vi "LabVIEW MIDI Keyboard.vi"() -> ()   [LabVIEW 2016]
doc: "This example simulates a General MIDI (GM) keyboard. Use the computer keys to play the general MIDI sound you select. The example uses Event structures to get the keyboard events and a Call Library Function Node to send the MIDI messages to Windows."
panel:
  in  "?":bool
  in  "Config":bool
  in  "Help":bool
  in  "stop":bool
  in  "General MIDI instrument patch":i32(listbox)
  in  "Volume":i32(knob)=110 min=0 max=127 step=1 scale=0.0..127.0
  in  "uDeviceID":i32=1
  in  "Midi channel":i32
  # "Select Help»Show Context Help and move the cursor over the VI icon to display help for this VI."
  # "Instructions:\n1. Run the VI.\n2. Select a sound type from the General MIDI instrument patch listbox.\n3. Press a key on the computer keyboard that corresponds to a key on the image of the MIDI keyboard.\n\nNOTE: If you do not hear a sound, click the Config button to change the MIDI device number. Refer to the Windows Device Manager to determine the correct MIDI device number.\n\n4. To stop the VI, click the Stop button or press the <Esc> key."
  # "Use myRio to get the note values ?"
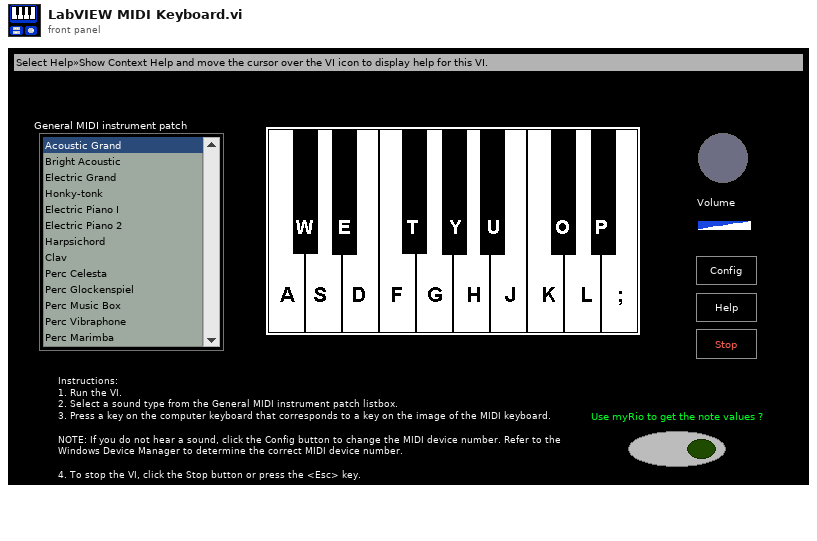
[diagram p1: front panel]
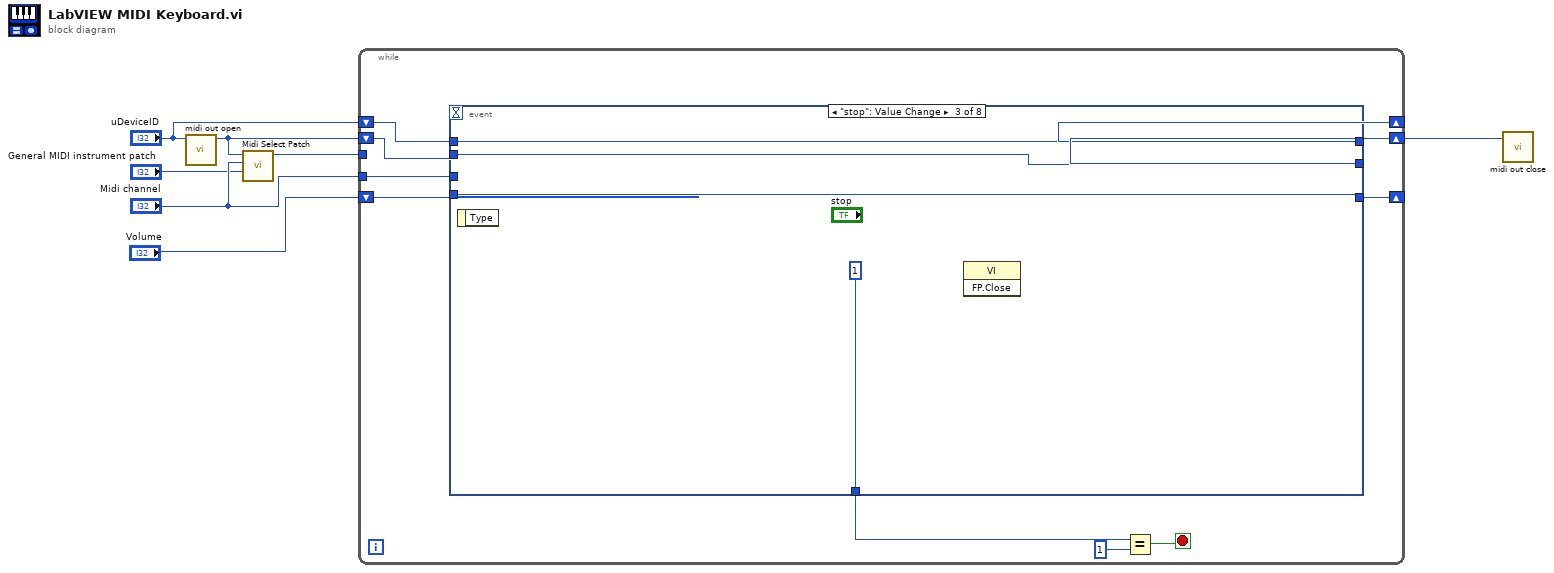
[diagram p0: block diagram]
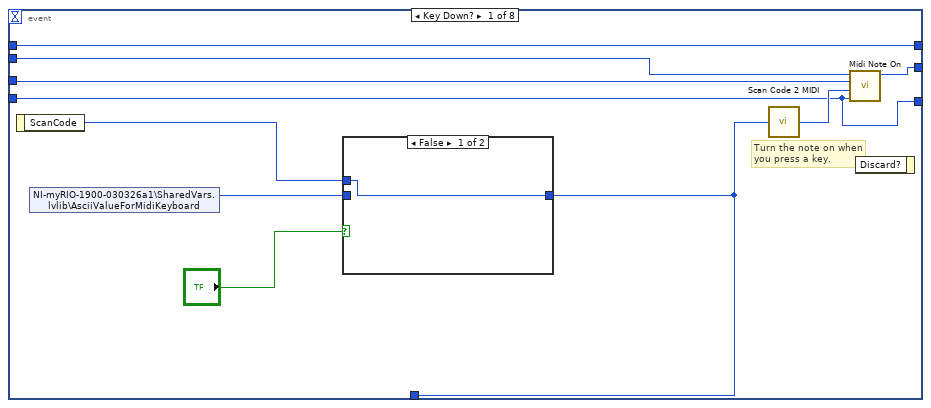
[diagram p2: hidden frame]
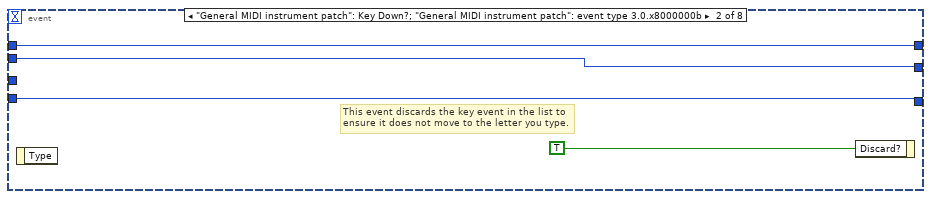
[diagram p4: hidden frame]
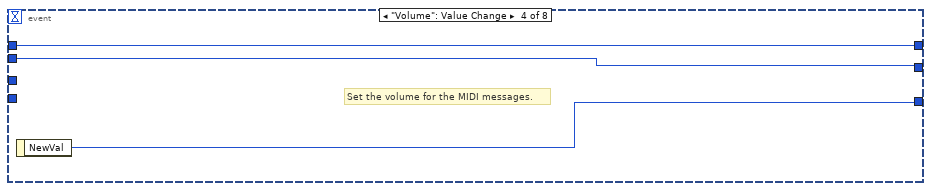
[diagram p5: hidden frame]
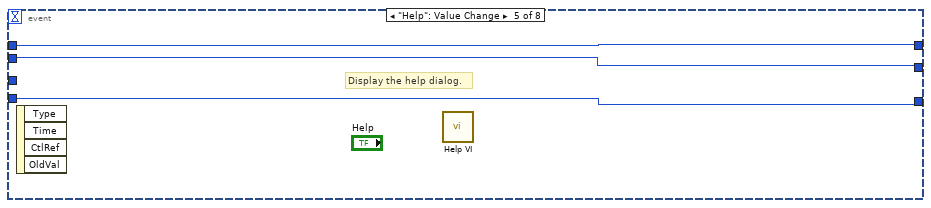
[diagram p6: hidden frame]
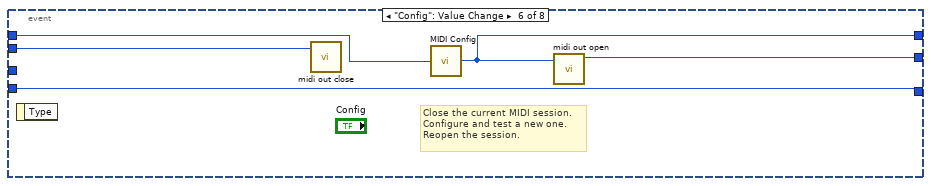
[diagram p7: hidden frame]
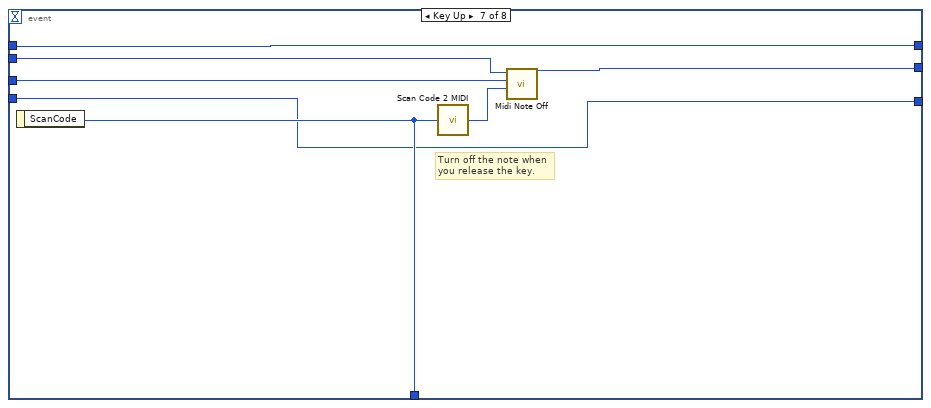
[diagram p8: hidden frame]
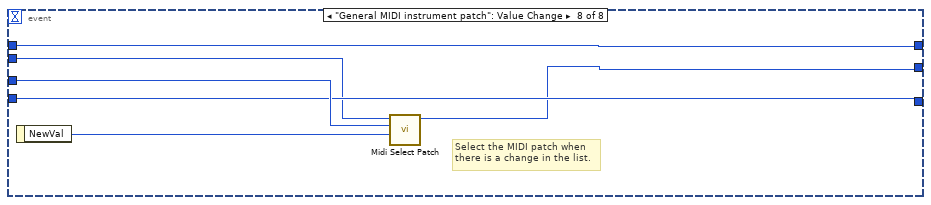
[diagram p9: hidden frame]
diagram:
  n1 = call "midi out open.vi"("UDeviceID"="uDeviceID") -> ("Hmidiout handle"=w3:i32)  [unwired: 5 in, 1 out]
  n2 = call "Midi Select Patch.vi"("Patch?"="General MIDI instrument patch", "Channel"="Midi channel", "MIDI out handle"=w3) -> ("Duplicate MIDI handle"=w7:i32)  [unwired: 3 in, 1 out]
  n3 = while {
    tunnel: w7 -> [_]
    tunnel: "Midi channel" -> [w17]
    shift-right: [w12] -> _
    shift-left: "Volume" -> [w13]
    shift-right: [w10] -> w2
    shift-left: w3 -> [w11]
    shift-right: [w8] -> _
    shift-left: "uDeviceID" -> [w9]
    stop <- w16 stop-if-true
    n4 = event shown="[2] \"stop\": Value Change" {
      selector: _ -> [_ _ _ _ _ _ _ _]
      dyn-events: _ -> [_ _ _ _ _ _ _ _]
      timeout: _ -> [_ _ _ _ _ _ _ _]
      tunnel: w11 -> [w22 w33 w37 w39 w42 w45 w50 w57]
      tunnel: w17 -> [w27 _ _ _ _ _ w55 w60]
      tunnel: w13 -> [w25 w32 w36 _ w43 w48 w52 w59]
      tunnel: [w23 w33 w37 w39 w42 w47 w49 w56] -> w10
      tunnel: [w18 _ i16 1 ("ScanCode") _ _ _ w53 _] -> w14
      tunnel: [w25 w32 w36 w40 w43 w48 w52 w59] -> w12
      tunnel: w9 -> [w24 w31 w35 w38 w41 w44 w51 w58]
      tunnel: [w24 w31 w35 w38 w41 w46 w51 w58] -> w8
      event Key Down? {
        # "Turn the note on when you press a key."
        n5 = event-data() -> ("ScanCode"=w19:i16)  [unwired: 1 in]
        n6 = shared-variable "NI-myRIO-1900-030326a1\\SharedVars.lvlib\\AsciiValueForMidiKeyboard"() -> (w20:i16)  [unwired: 1 in, 1 out]
        n7 = case shown="False" "?" {
          tunnel: w20 -> [_ w29]
          tunnel: w19 -> [w28 _]
          tunnel: [w28 w29] -> w18
          frame False {
          }
          frame True {
          }
        }
        n8 = call "Scan Code 2 MIDI.vi"("ScanCode"=w18) -> ("MIDI note"=w26:i32)  [unwired: 4 in]
        n9 = call "Midi Note On.vi"("Volume"=w25, "Note"=w26, "Channel"=w27, "MIDI handle"=w22) -> ("Duplicate MIDI handle"=w23:i32)  [unwired: 2 in, 1 out]
        n10 = event-data() -> ()  [unwired: 2 in, 1 out]
      }
      event "General MIDI instrument patch": Key Down?; "General MIDI instrument patch": event type 3.0.x8000000b {
        # "This event discards the key event in the list to ensure it does not move to the letter you type."
        n11 = event-data() -> ()  [unwired: 1 in, 1 out]
        n12 = event-data("Discard?"=TRUE) -> ()  [unwired: 1 in, 1 out]
      }
      event "stop": Value Change {
        n13 = event-data() -> ()  [unwired: 1 in, 1 out]
        n14 = invoke class="VI" method="FP.Close"() -> ()  [unwired: 3 in, 3 out]
      }
      event "Volume": Value Change {
        # "Set the volume for the MIDI messages."
        n15 = event-data() -> ("NewVal"=w40:i32)  [unwired: 1 in]
      }
      event "Help": Value Change {
        # "Display the help dialog."
        n16 = event-data() -> ()  [unwired: 1 in, 4 out]
        n17 = call "Help VI.vi"() -> ()  [unwired: 1 in]
      }
      event "Config": Value Change {
        # "Close the current MIDI session.\nConfigure and test a new one.\nReopen the session."
        n18 = event-data() -> ()  [unwired: 1 in, 1 out]
        n19 = call "midi out close.vi"("MIDI output handle"=w45) -> ()  [unwired: 6 in, 1 out]
        n20 = call "MIDI Config.vi"("MIDI device:"=w44) -> ("Selected device"=w46:i32)  [unwired: 4 in]
        n21 = call "midi out open.vi"("UDeviceID"=w46) -> ("Hmidiout handle"=w47:i32)  [unwired: 5 in, 1 out]
      }
      event Key Up {
        # "Turn off the note when you release the key."
        n22 = event-data() -> ("ScanCode"=w53:i16)  [unwired: 1 in]
        n23 = call "Scan Code 2 MIDI.vi"("ScanCode"=w53) -> ("MIDI note"=w54:i32)  [unwired: 4 in]
        n24 = call "Midi Note Off.vi"("Note"=w54, "Channel"=w55, "MIDI handle"=w50) -> ("Duplicate MIDI handle"=w49:i32)  [unwired: 3 in, 1 out]
      }
      event "General MIDI instrument patch": Value Change {
        # "Select the MIDI patch when\nthere is a change in the list."
        n25 = event-data() -> ("NewVal"=w61:i32)  [unwired: 1 in]
        n26 = call "Midi Select Patch.vi"("Patch?"=w61, "Channel"=w60, "MIDI out handle"=w57) -> ("Duplicate MIDI handle"=w56:i32)  [unwired: 3 in, 1 out]
      }
    }
    n27 = Equal?(x=w14, y=i16 1) -> (x = y?=w16:bool)
  }
  n28 = call "midi out close.vi"("MIDI output handle"=w2) -> ()  [unwired: 6 in, 1 out]
